vi "I2C.Read.vi"(5 "I2C Address":u16 format="%x", 7 "I2C Register":u16 format="%x", 8 "error in":errorcluster, 9 "Read/Write Mode":T1(ring), 10 "I2C Write Data":u8[](array[numeric]), 11 "comport in":refnum<visa-resource-name>) -> (0 "error out":errorcluster={"status"=TRUE, "code"=-1073807339, "source"="VISA Read in FirmataClient.lvlib:Initialize.vi"}, 1 "I2CDataAsASCII":string, 2 "I2CDataAsArray":u8[](array[numeric]), 3 "comport out":refnum<visa-resource-name>, 4 "I2C Address Out":u8 format="%x", 6 "I2C Register Out":u64 format="%x")   [LabVIEW 2020, in "FirmataClient.lvlib"]
doc: "Reads a string from a UUT's target I2C device running on its board"
uses:
  FirmataClient.lvlib
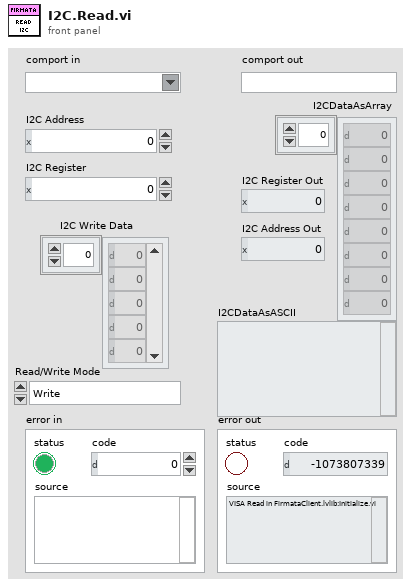
[diagram p1: front panel]
types:
  T1 = enum16{"Write", "Read Once", "Read Continuously", "Stop Continuous Reading"}
  T2 = typedef "FirmataClient.lvlib/FirmataProtocolConstants.ctl" = u16
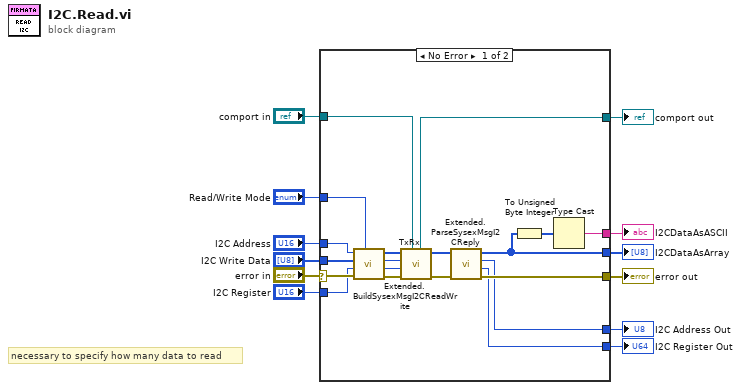
[diagram p0: block diagram]
diagram:
  # "necessary to specify how many data to read"
  n1 = case shown="No Error" "error in" {
    selector: "error in" -> [w25 w33]
    tunnel: [w22 w33] -> w11
    tunnel: [w27 w32] -> w2
    tunnel: "comport in" -> [w26 w32]
    tunnel: "Read/Write Mode" -> [w13 _]
    tunnel: "I2C Address" -> [w19 _]
    tunnel: "I2C Write Data" -> [w15 _]
    tunnel: [w17 _] -> w6
    tunnel: [w21 _] -> w5
    tunnel: [w20 _] -> w4
    tunnel: "I2C Register" -> [w14 _]
    tunnel: [w18 _] -> w1
    frame No Error {
      n2 = call "Extended.BuildSysexMsgI2CReadWrite.vi"("Read/Write Mode"=w13, "error in"=w25, "Register"=w14, "I2C Write Data"=w15, "Slave Address"=w19) -> ("error out"=w31:errorcluster, "ReplyLength"=w28:i32, "ReplyFirstByte"=w29:T2, "I2CRequestMessage"=w30:u8[])  [unwired: 3 in]
      n3 = call "TxRx.vi"("comport in"=w26, "error in"=w31, "Expected Reply Length"=w28, "ReplyFirstByte"=w29, "MessageToSend"=w30) -> ("error out"=w24:errorcluster, "ReceivedMessage"=w23:u8[], "comport out"=w27:refnum<visa-resource-name>)  [unwired: 2 in, 2 out]
      n4 = call "Extended.ParseSysexMsgI2CReply.vi"("error in"=w24, "Sysex Message"=w23) -> ("error out"=w22:errorcluster, "I2C Register"=w20:u64, "I2C Address"=w21:u8, "I2C Data"=w17:u16[])  [unwired: 6 in]
      n5 = To Unsigned Byte Integer(number=w17) -> (unsigned 8bit integer=w16:u8[])
      n6 = Type Cast(x=w16) -> (*(type *) &x=w18:string)  [unwired: 1 in]
    }
    frame Error {
    }
  }
  "error out" <- w11
  "I2CDataAsArray" <- w6
  "I2C Address Out" <- w5
  "I2C Register Out" <- w4
  "comport out" <- w2
  "I2CDataAsASCII" <- w1
